vi "Turn On-Off 5V.vi"(8 "error in (no error)":errorcluster, 10 "Value":bool=TRUE, 11 "I-O in":refnum<class "I-O.lvclass">) -> (0 "error out":errorcluster, 3 "I-O out":refnum<class "I-O.lvclass">)   [LabVIEW 2021, in "I-O.lvclass"]
uses:
  I-O.lvclass
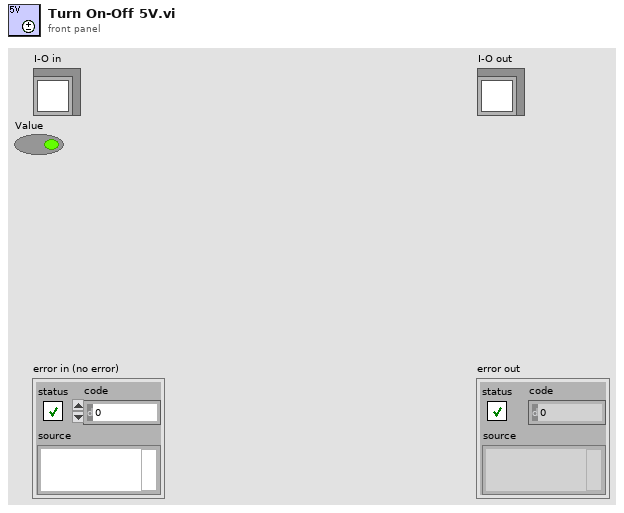
[diagram p1: front panel]
types:
  T1 = typedef "I-O.lvclass/Pin Map.ctl" = cluster{"Region Valves":i32[], "Extra Valves":dbl[][][], "Tool Primary Valve":i32, "Tool Secondary Valve":i32, "Region Sensors":i32[], "Extra Sensors":dbl[][][], "Tool Primary Sensor":dbl, "Tool Secondary Sensor":dbl, "Compression Sensor":dbl, "5V":i32, "Dispenser Sensor":dbl, "Light Curtain":i32}
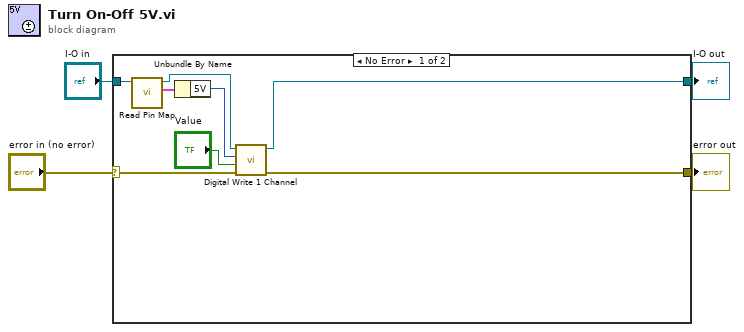
[diagram p0: block diagram]
diagram:
  n1 = case shown="No Error" "error in (no error)" {
    selector: "error in (no error)" -> [w11 w14]
    tunnel: [w10 w14] -> w3
    tunnel: [w12 w13] -> w1
    tunnel: "I-O in" -> [w9 w13]
    frame No Error {
      n2 = call-dynamic "Read Pin Map.vi"("I-O in"=w9) -> ("Pin Map 2"=w6:T1, "I-O out"=w5:refnum<class "I-O.lvclass">)  [unwired: 8 in, 1 out]
      n3 = Unbundle By Name(w6) -> ("5V"=w7:i32)
      n4 = call-dynamic "Digital Write 1 Channel.vi"("error constant"=w11, "Value"="Value", "Channel"=w7, "I-O.lvclass"=w5) -> ("error IO"=w10:errorcluster, "I-O.lvclass 2"=w12:refnum<class "I-O.lvclass">)  [unwired: 6 in]
    }
    frame Error {
    }
  }
  "error out" <- w3
  "I-O out" <- w1
